vi "Untitled 1.vi"() -> ()   [LabVIEW 2020]
panel:
  in  "Simulate Pill Drop":bool
  out "Waveform Chart":dbl(graph)
  out "Temperature":dbl
  out "Pill Count":dbl
  out "DAQ Voltage":dbl
  out "Fan Trigger":bool
  out "Ready to Dispense":bool
  out "Temp Safe":bool
  out "Bottle Present":bool
  in  "Humidity":dbl(knob) scale=0.0..100.0
  in  "Temperature(C)":dbl(knob) scale=20.0..70.0 scale format="%#_2g"
  in  "Bottle Weight(g)":dbl(slide) scale=0.0..500.0
  in  "stop":bool
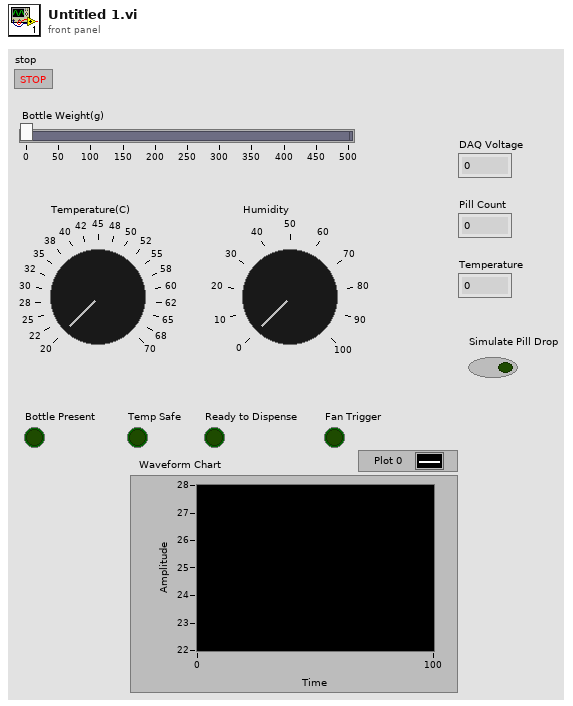
[diagram p1: front panel]
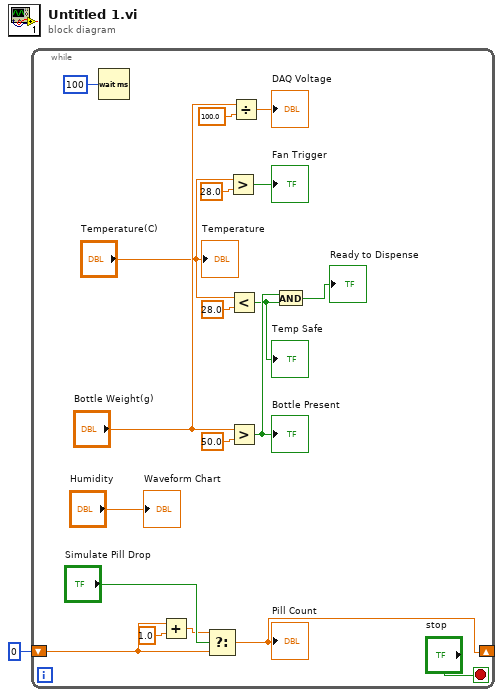
[diagram p0: block diagram]
diagram:
  n1 = while {
    shift-right: [w2] -> _
    shift-left: 0 -> [w3]
    stop <- "stop" stop-if-true
    n2 = Wait (ms)(milliseconds to wait=u32 100) -> ()  [unwired: 1 out]
    n3 = Add(x=w3, y=1.0) -> (x+y=w4:dbl)
    n4 = Select(t=w4, s="Simulate Pill Drop", f=w3) -> (s? t:f=w2:dbl)
    "Pill Count" <- w2
    n5 = Greater?(x="Temperature(C)", y=28.0) -> (0:→"Fan Trigger":bool)
    n6 = Less?(x="Temperature(C)", y=28.0) -> (x < y?=w10:bool)
    "Temp Safe" <- w10
    n7 = Greater?(x="Bottle Weight(g)", y=50.0) -> (0:w11:bool)
    "Bottle Present" <- w11
    n8 = Divide(x="Bottle Weight(g)", y=100.0) -> (x/y=→"DAQ Voltage":dbl)
    n9 = And(x=w11, y=w10) -> (x .and. y?=→"Ready to Dispense":bool)
    "Temperature" <- "Temperature(C)"
    "Waveform Chart" <- "Humidity"
  }
